vi "LitePoint_QueryandReset.vi"(8 "error in (no error)":errorcluster, 9 "Reset (True)":bool=TRUE, 10 "ID Query (True)":bool=TRUE, 11 "VISA resource name":refnum<visa-resource-name>) -> (0 "error out":errorcluster, 2 "read buffer":string, 3 "VISA resource name out":refnum<visa-resource-name>)   [LabVIEW 2020, in "LitePoints.lvlib"]
uses:
  LitePoints.lvlib
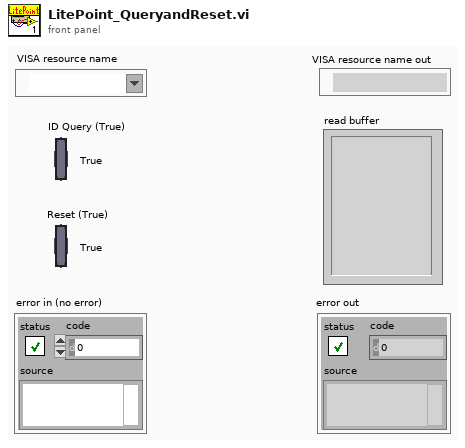
[diagram p1: front panel]
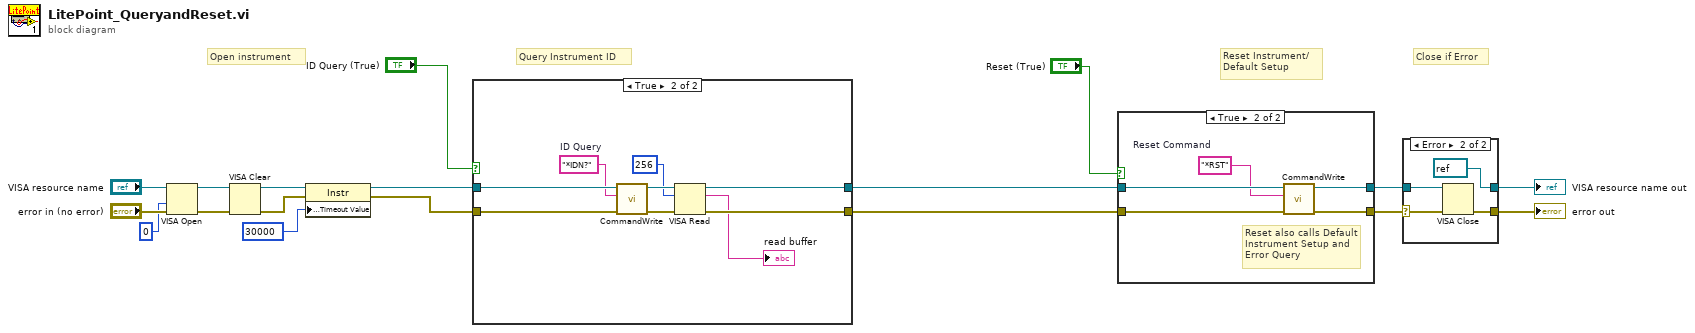
[diagram p0: block diagram]
diagram:
  # "Close if Error"
  # "Query Instrument ID"
  # "Reset Instrument/\nDefault Setup"
  # "Open instrument"
  n1 = VISA Open(access mode=u32 0, error in (no error)="error in (no error)", VISA resource name="VISA resource name") -> (VISA resource name=w12:refnum<visa-resource-name>, error out=w11:errorcluster)  [unwired: 2 out]
  n2 = VISA Clear(VISA resource name=w12, error in (no error)=w11) -> (VISA resource name out=w10:refnum<visa-resource-name>, error out=w9:errorcluster)
  n3 = property class="Instr"(reference=w10, error in=w9, "General Settings:Timeout Value"=u32 30000) -> (reference out=w4:refnum<visa-resource-name>, error out=w3:errorcluster)
  n4 = case shown="True" "ID Query (True)" {
    tunnel: [w19 w22] -> w1
    tunnel: [w20 w27] -> w2
    tunnel: w4 -> [w20 w28]
    tunnel: w3 -> [w19 w29]
    frame False {
    }
    frame True {
      w23 = "*IDN?"  # ID Query
      n5 = call "CommandWrite.vi"("error in (no error)"=w29, "Write Buffer"=w23, "VISA resource name"=w28) -> ("error out"=w25:errorcluster, "VISA resource name out"=w26:refnum<visa-resource-name>)  [unwired: 7 in]
      n6 = VISA Read(VISA resource name=w26, byte count=u32 256, error in (no error)=w25) -> (VISA resource name out=w27:refnum<visa-resource-name>, read buffer=→"read buffer":string, error out=w22:errorcluster)  [unwired: 1 out]
    }
  }
  n7 = case shown="True" "Reset (True)" {
    tunnel: [w30 w36] -> w5
    tunnel: [w31 w35] -> w6
    tunnel: w2 -> [w31 w34]
    tunnel: w1 -> [w30 w33]
    frame False {
    }
    frame True {
      w32 = "*RST"  # Reset Command
      # "Reset also calls Default Instrument Setup and Error Query"
      n8 = call "CommandWrite.vi"("error in (no error)"=w33, "Write Buffer"=w32, "VISA resource name"=w34) -> ("error out"=w36:errorcluster, "VISA resource name out"=w35:refnum<visa-resource-name>)  [unwired: 7 in]
    }
  }
  n9 = case shown="Error" w5 {
    selector: w5 -> [w37 w40]
    tunnel: w6 -> [w38 w41]
    tunnel: [w38 refnum<visa-resource-name> refnum ("VISA resource name out")] -> w8
    tunnel: [w37 w39] -> w7
    frame No Error {
    }
    frame Error {
      n10 = VISA Close(VISA resource name=w41, error in (no error)=w40) -> (error out=w39:errorcluster)
    }
  }
  "VISA resource name out" <- w8
  "error out" <- w7
